vi "Data File Processing UI Manager.vi"(7 "Method":T3=enum."SendMSG", 9 "data":variant, 10 "msg type":T1=enum."NoEvent") -> ()   [LabVIEW 2012]
doc: "This VI maintains the list of host connections."
uses:
  Data File Processing UI Manager.ctl
  Data File Processing UI Message Define.ctl
  Data File Processing UI Message Type Define.ctl
panel:
  in  "temp msg def":T2
  in  "error in":errorcluster
  out "error out":errorcluster
  # "Input Data"
  # "Local Data"
  # "Output Data"
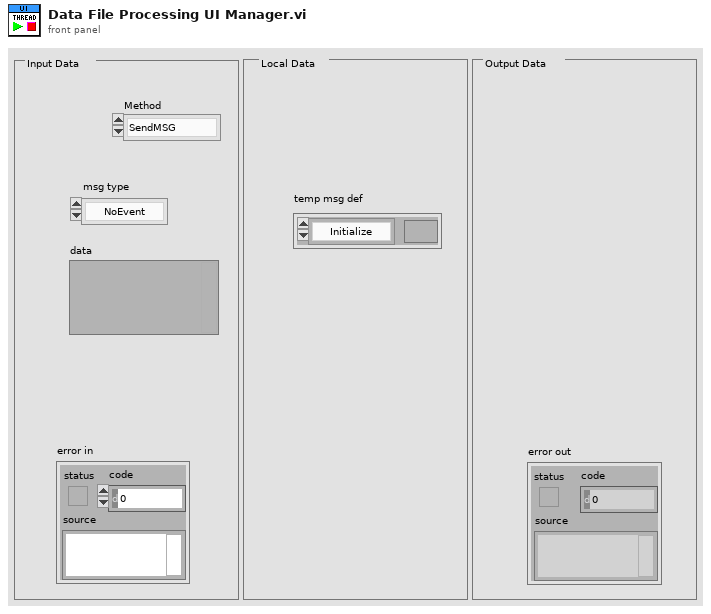
[diagram p1: front panel]
types:
  T1 = typedef "Data File Processing UI Message Type Define.ctl" = enum32{"Initialize", "SleepThread", "ErrorHandler", "NoEvent", "PreExit", "Exit", "----Action----", "OpenFile", "ReadAllCompute", "SaveFile", "RedrawGraph", "SelectChannel"}
  T2 = typedef "Data File Processing UI Message Define.ctl" = cluster{"data":variant, "type":T1}
  T3 = typedef "Data File Processing UI Manager.ctl" = enum16{"Create", "SendMSG", "Close"}
  T4 = enum32{"Invalid", "Standard", "Closed", "Hidden", "Minimized", "Maximized"}
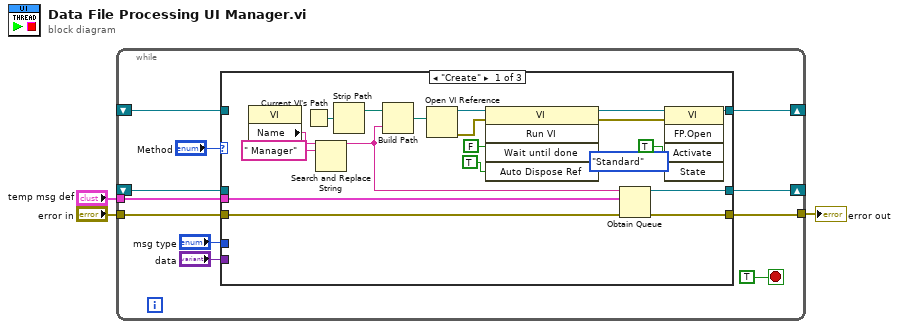
[diagram p0: block diagram]
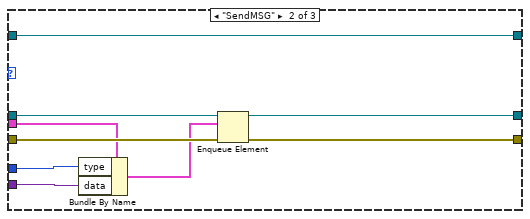
[diagram p2: hidden frame]
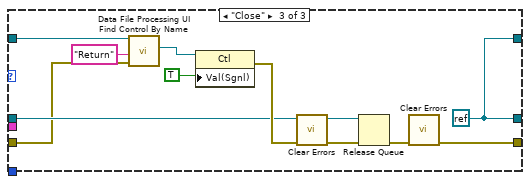
[diagram p3: hidden frame]
diagram:
  n1 = while {
    tunnel: "error in" -> [w12]
    tunnel: [w9] -> w2
    shift-right: [w10] -> _
    shift-left: _ -> [w11]
    tunnel: "temp msg def" -> [w8]
    shift-right: [w6] -> _
    shift-left: _ -> [w5]
    stop <- TRUE stop-if-true
    n2 = case shown="\"Create\"" "Method" {
      tunnel: [w31 w39 w48] -> w9
      tunnel: w12 -> [w33 w40 w46]
      tunnel: [w32 w41 w50] -> w10
      tunnel: w11 -> [_ w42 w51]
      tunnel: "msg type" -> [_ w38 _]
      tunnel: "data" -> [_ w37 _]
      tunnel: w8 -> [w30 w35 _]
      tunnel: [w19 w34 w50] -> w6
      tunnel: w5 -> [_ w34 w47]
      frame "Create" {
        n3 = property class="VI"() -> ("Name"=w28:string)  [unwired: 2 in, 2 out]
        n4 = Current VI's Path() -> (path=w20:path)
        n5 = Search and Replace String(input string=w28, search string=" Manager") -> (result string=w15:string)  [unwired: 6 in, 3 out]
        n6 = Strip Path(path=w20) -> (stripped path=w16:path)  [unwired: 1 out]
        n7 = Build Path(base path=w16, name or relative path=w15) -> (appended path=w21:path)
        n8 = Open VI Reference(vi path=w21) -> (vi reference=w18:refnum<vi>, error out=w17:errorcluster)  [unwired: 5 in]
        n9 = invoke class="VI" method="Run VI"(reference=w18, error in=w17, "Wait until done"=FALSE, "Auto Dispose Ref"=TRUE) -> (reference out=w25:refnum<vi>, error out=w24:errorcluster)  [unwired: 1 in, 3 out]
        n10 = Obtain Queue(name (unnamed)=w15, element data type=w30, error in (no error)=w33) -> (queue out=w32:refnum<queue>, error out=w31:errorcluster)  [unwired: 2 in, 1 out]
        n11 = invoke class="VI" method="FP.Open"(reference=w25, error in=w24, "Activate"=TRUE, "State"=T4."Standard" ("FP state")) -> (reference out=w19:refnum<vi>)  [unwired: 1 in, 4 out]
      }
      frame "SendMSG" {
        n12 = Bundle By Name(cluster=w35, "type"=w38, "data"=w37) -> (w36:T2)
        n13 = Enqueue Element(queue=w42, element=w36, error in (no error)=w40) -> (queue out=w41:refnum<queue>, error out=w39:errorcluster)  [unwired: 1 in, 1 out]
      }
      frame "Close" {
        w50 = refnum<k0> refnum
        n14 = call "Data File Processing UI Find Control By Name.vi"("error in (no error)"=w46, "control name"="Return" ("Control Name"), "vi refnum in"=w47) -> ("control refnum"=w44:refnum<vi>)  [unwired: 6 in, 2 out]
        n15 = property class="Ctl"(reference=w44, "Val(Sgnl)"=TRUE ("force destroy? (F)")) -> (error out=w53:errorcluster)  [unwired: 1 in, 1 out]
        n16 = call <vilib>:"Clear Errors.vi"("error in (no error)"=w53) -> ("error out"=w52:errorcluster)  [unwired: 6 in]
        n17 = Release Queue(queue=w51, error in (no error)=w52) -> (error out=w49:errorcluster)  [unwired: 1 in, 2 out]
        n18 = call <vilib>:"Clear Errors.vi"("error in (no error)"=w49) -> ("error out"=w48:errorcluster)  [unwired: 6 in]
      }
    }
  }
  "error out" <- w2
